vi "ALU.vi"(11 "ALU Inputs":T1) -> (0 "MulOut":dbl, 1 "SubOut":dbl, 2 "AddOut":dbl, 3 "DivOut":dbl)   [LabVIEW 2020]
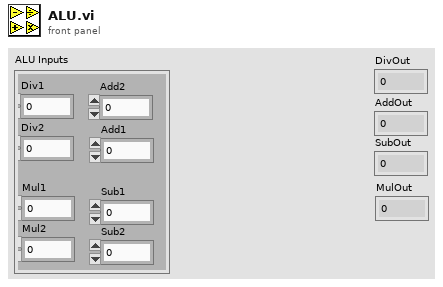
[diagram p1: front panel]
types:
  T1 = cluster{"Div1":dbl, "Div2":dbl, "Add1":dbl, "Add2":dbl, "Sub1":dbl, "Sub2":dbl, "Mul1":dbl, "Mul2":dbl}
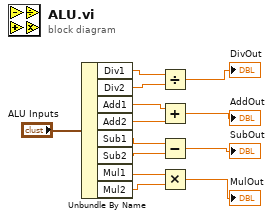
[diagram p0: block diagram]
diagram:
  n1 = Unbundle By Name("ALU Inputs") -> ("Div1"=w12:dbl, "Div2"=w11:dbl, "Add1"=w10:dbl, "Add2"=w9:dbl, "Sub1"=w8:dbl, "Sub2"=w7:dbl, "Mul1"=w6:dbl, "Mul2"=w5:dbl)
  n2 = Divide(x=w12, y=w11) -> (x/y=→"DivOut":dbl)
  n3 = Add(x=w10, y=w9) -> (x+y=→"AddOut":dbl)
  n4 = Subtract(x=w8, y=w7) -> (x-y=→"SubOut":dbl)
  n5 = Multiply(x=w6, y=w5) -> (x*y=→"MulOut":dbl)
